vi "Extract Single Tone Information from Hann Spectrum.vi"(0 "complex spectrum in":cdb[](array[numeric]) format="%0.2f", 1 "time signal in":dbl[](array[numeric]) format="%0.2f", 5 "FFT size":i32, 7 "export mode":T2(ring), 9 "sampling frequency":dbl format="%0.2f", 11 "error in":errorcluster, 12 "advanced search":T3={"approx freq. (optional)"=-1.0, "search (+/- % of Fsampl.)"=5.0} {"search (+/- % of Fsampl.)" format="%0.2f"; "approx freq. (optional)" format="%0.2f"}) -> (3 "time signal out":dbl[](array[numeric]) format="%0.2p", 4 "complex spectrum out":cdb[](array[numeric]) format="%0.2f", 6 "detected frequency":dbl format="%0.3p", 8 "detected amplitude":dbl format="%0.3p", 10 "detected phase (deg)":dbl format="%0.3p", 14 "measurement info":T1 {"uncertainty" format="%0.2p"}, 15 "error out":errorcluster)   [LabVIEW 2020, in "NI_MAPro.lvlib"]
uses:
  NI_MAPro.lvlib
  NI_AALBase.lvlib
panel:
  # "Extract Single Tone Information\nfrom Hann weighted Spectrum"
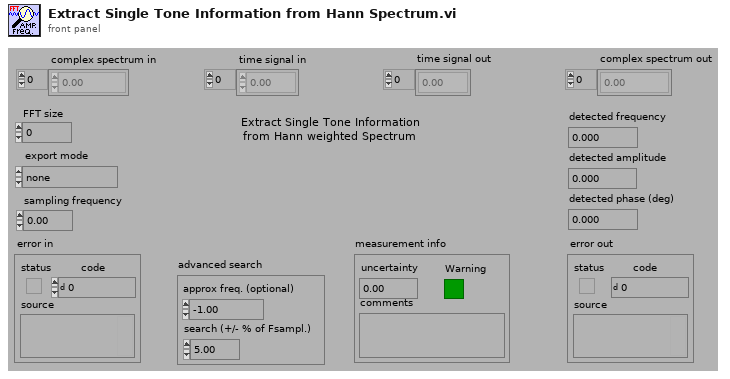
[diagram p1: front panel]
types:
  T1 = cluster{"uncertainty":dbl, "Warning":bool, "comments":string}
  T2 = enum32{"none", "input signal", "detected signal", "residual signal"}
  T3 = cluster{"approx freq. (optional)":dbl, "search (+/- % of Fsampl.)":dbl}
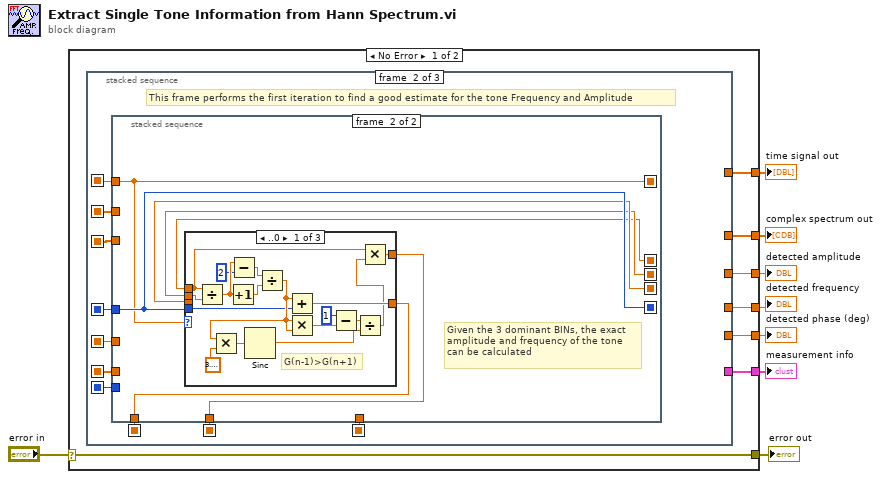
[diagram p0: block diagram]
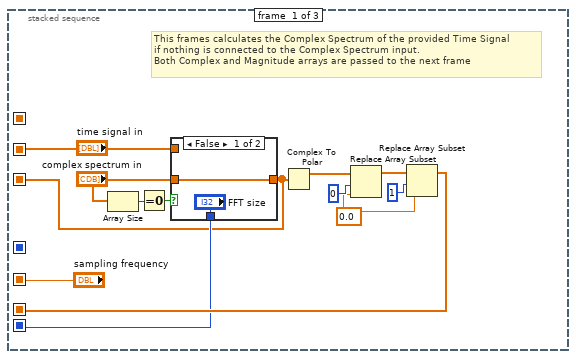
[diagram p2: hidden frame]
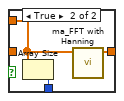
[diagram p3: hidden frame]
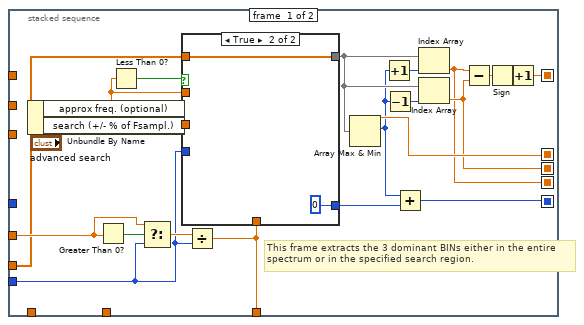
[diagram p4: hidden frame]
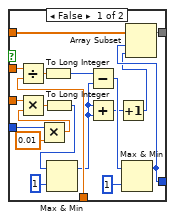
[diagram p5: hidden frame]
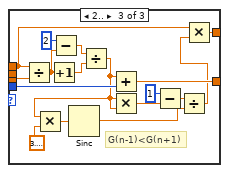
[diagram p7: hidden frame]
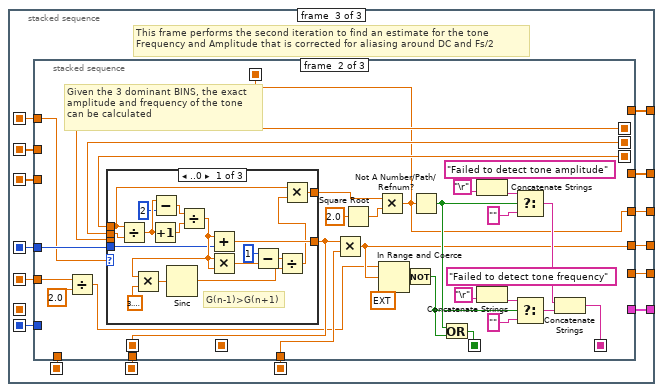
[diagram p8: hidden frame]
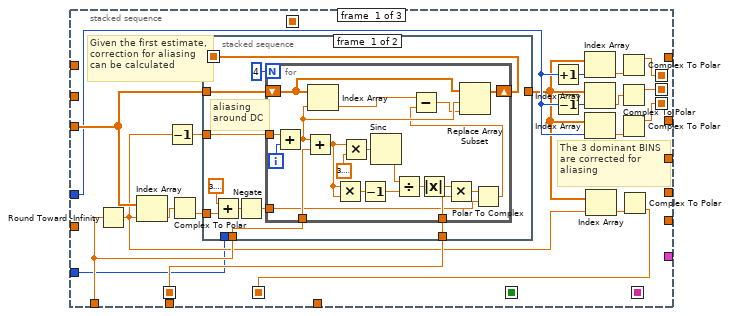
[diagram p9: hidden frame]
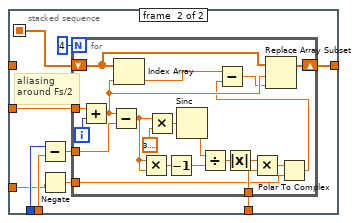
[diagram p10: hidden frame]
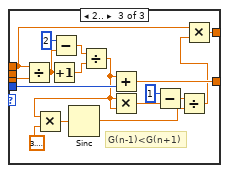
[diagram p12: hidden frame]
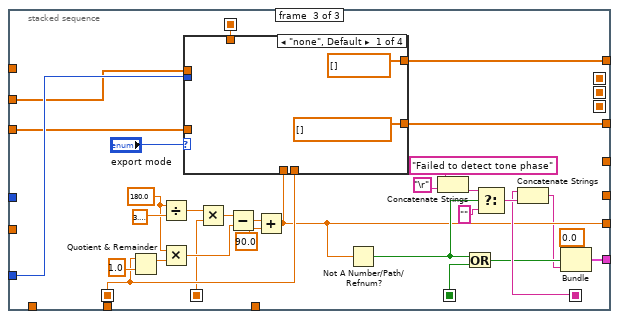
[diagram p13: hidden frame]
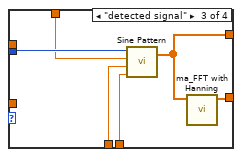
[diagram p15: hidden frame]
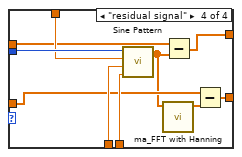
[diagram p16: hidden frame]
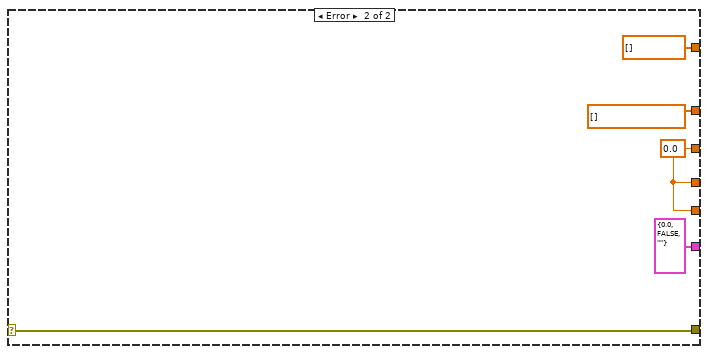
[diagram p17: hidden frame]
diagram:
  n1 = case shown="No Error" "error in" {
    selector: "error in" -> [w9 w343]
    tunnel: [w9 w343] -> w8
    tunnel: [w15 dbl[] [] ("Sinusoidal Pattern")] -> w7
    tunnel: [w14 cdb[] [] ("complex spectrum")] -> w6
    tunnel: [w13 w345] -> w5
    tunnel: [w12 w345] -> w4
    tunnel: [w11 w345] -> w3
    tunnel: [w10 cluster{dbl, bool, string} {0.0, FALSE, ""}] -> w2
    frame No Error {
      n2 = stacked-sequence {
        seq-local: ["time signal in" _ _] -> [_ w43 w140]
        seq-local: [w16 _ _] -> [_ w42 w139]
        seq-local: ["sampling frequency" _ _] -> [_ w41 w130]
        seq-local: [w25 _ _] -> [_ w40 _]
        seq-local: [w24 _ _] -> [_ w39 w141]
        seq-local: [_ w38 _] -> [_ _ w138]
        seq-local: [_ w37 _] -> [_ _ w143]
        seq-local: [_ w36 _] -> [_ _ w144]
        seq-local: [_ w35 _] -> [_ _ w137]
        seq-local: [_ w34 _] -> [_ _ w142]
        tunnel: [_ _ w136] -> w15
        tunnel: [_ _ w135] -> w14
        tunnel: [_ _ w134] -> w13
        tunnel: [_ _ w133] -> w12
        tunnel: [_ _ w132] -> w11
        tunnel: [_ _ w131] -> w10
        frame #0 {
          w20 = 0.0
          # "This frames calculates the Complex Spectrum of the provided Time Signal\nif nothing is connected to the Complex Spectrum input.\nBoth Complex and Magnitude arrays are passed to the next frame"
          n3 = Array Size(array="complex spectrum in") -> (size(s)=w18:i32)
          n4 = Equal To 0?(x=w18) -> (x = 0?=w17:bool)
          n5 = case shown="False" w17 {
            tunnel: [w30 w33] -> w16
            tunnel: "complex spectrum in" -> [w30 _]
            tunnel: "time signal in" -> [_ w32]
            tunnel: ["FFT size" w31] -> w24
            frame False {
            }
            frame True {
              n6 = Array Size(array=w32) -> (size(s)=w31:i32)
              n7 = call "ma_FFT with Hanning.vi"("time signal data"=w32) -> ("complex Hann spectrum"=w33:cdb[])  [unwired: 2 in, 8 out]
            }
          }
          n8 = Complex To Polar(r * e^(i*theta)=w16) -> (r=w23:dbl[])  [unwired: 1 out]
          n9 = Replace Array Subset(array=w23, new element=w20, index=0) -> (w22:dbl[])
          n10 = Replace Array Subset(array=w22, new element=w20, index=1) -> (w25:dbl[])
        }
        frame #1 {
          # "This frame performs the first iteration to find a good estimate for the tone Frequency and Amplitude"
          n11 = stacked-sequence {
            seq-local: [w58 _] -> [_ w90]
            seq-local: [w57 _] -> [_ w91]
            seq-local: [w56 _] -> [_ w92]
            seq-local: [w45 _] -> [_ w93]
            seq-local: [w55 _] -> [_ w87]
            tunnel: w43 -> [_ _]
            tunnel: w42 -> [_ _]
            tunnel: w41 -> [w50 _]
            tunnel: w40 -> [w49 _]
            tunnel: w39 -> [w48 _]
            tunnel: [_ w89] -> w38
            tunnel: [_ w93] -> w37
            tunnel: [w47 _] -> w36
            tunnel: [_ w88] -> w35
            tunnel: [_ w87] -> w34
            frame #0 {
              # "This frame extracts the 3 dominant BINs either in the entire\nspectrum or in the specified search region."
              n12 = Unbundle By Name("advanced search") -> ("approx freq. (optional)"=w52:dbl, "search (+/- % of Fsampl.)"=w65:dbl)
              n13 = Greater Than 0?(x=w50) -> (x > 0?=w53:bool)
              n14 = Less Than 0?(x=w52) -> (x < 0?=w63:bool)
              n15 = Select(t=w50, s=w53, f=w48) -> (s? t:f=w54:dbl)
              n16 = Divide(x=w54, y=w48) -> (x/y=w47:dbl)
              n17 = case shown="True" w63 {
                tunnel: [w74 w86] -> w64
                tunnel: w49 -> [w76 w86]
                tunnel: w48 -> [w84 _]
                tunnel: w65 -> [w82 _]
                tunnel: w47 -> [w79 _]
                tunnel: w52 -> [w80 _]
                tunnel: [w72 0] -> w44
                frame False {
                  n18 = Divide(x=w80, y=w79) -> (x/y=w78:dbl)
                  n19 = Multiply(x=w84, y=0.01) -> (x*y=w81:dbl)
                  n20 = Multiply(x=w82, y=w81) -> (x*y=w77:dbl)
                  n21 = To Long Integer(number=w78) -> (32bit integer=w75:i32)
                  n22 = To Long Integer(number=w77) -> (32bit integer=w67:i32)
                  n23 = Max & Min(x=w67, y=1 ("x")) -> (max(x,y)=w66:i32)  [unwired: 1 out]
                  n24 = Subtract(x=w75, y=w66) -> (x-y=w73:i32)
                  n25 = Add(x=w66, y=w66) -> (x+y=w70:i32)
                  n26 = Increment(x=w70) -> (x+1=w69:i32)
                  n27 = Max & Min(x=w73, y=1) -> (max(x,y)=w72:i32)  [unwired: 1 out]
                  n28 = Array Subset(array=w76, index=w72, length=w69) -> (w74:dbl[])
                }
                frame True {
                }
              }
              n29 = Array Max & Min(array=w64) -> (max value=w58:dbl, max index (indices)=w46:i32)  [unwired: 2 out]
              n30 = Increment(x=w46) -> (x+1=w59:i32)
              n31 = Decrement(x=w46) -> (x-1=w60:i32)
              n32 = Add(x=w46, y=w44) -> (x+y=w45:i32)
              n33 = Index Array(array=w64, index=w59) -> (element=w56:dbl)
              n34 = Index Array(array=w64, index=w60) -> (element=w57:dbl)
              n35 = Subtract(x=w56, y=w57) -> (x-y=w61:dbl)
              n36 = Sign(1:w61) -> (0:w62:dbl)
              n37 = Increment(x=w62) -> (x+1=w55:dbl)
            }
            frame #1 {
              # "Given the 3 dominant BINs, the exact\namplitude and frequency of the tone\ncan be calculated"
              n38 = case shown="..0" w87 {
                tunnel: w92 -> [_ _ w115]
                tunnel: w91 -> [w110 _ _]
                tunnel: w90 -> [w99 w111 w116]
                tunnel: [w107 w112 w125] -> w89
                tunnel: [w101 w111 w118] -> w88
                tunnel: w93 -> [w95 w112 w124]
                frame ..0 {
                  # "G(n-1)>G(n+1)"
                  n39 = Divide(x=w99, y=w110) -> (x/y=w97:dbl)
                  n40 = Increment(x=w97) -> (x+1=w108:dbl)
                  n41 = Subtract(x=w97, y=2) -> (x-y=w109:dbl)
                  n42 = Divide(x=w109, y=w108) -> (x/y=w104:dbl)
                  n43 = Multiply(x=w104, y=3.141592653589793) -> (x*y=w98:dbl)
                  n44 = Sinc(1:w98) -> (0:w94:dbl)
                  n45 = Add(x=w104, y=w95) -> (x+y=w107:dbl)
                  n46 = Multiply(x=w104, y=w104) -> (x*y=w103:dbl)
                  n47 = Subtract(x=1, y=w103) -> (x-y=w102:dbl)
                  n48 = Divide(x=w102, y=w94) -> (x/y=w100:dbl)
                  n49 = Multiply(x=w99, y=w100) -> (x*y=w101:dbl)
                }
                frame 1 {
                  # "G(n-1)=G(n+1)"
                }
                frame 2.. {
                  # "G(n-1)<G(n+1)"
                  n50 = Divide(x=w116, y=w115) -> (x/y=w128:dbl)
                  n51 = Increment(x=w128) -> (x+1=w126:dbl)
                  n52 = Subtract(x=2, y=w128) -> (x-y=w127:dbl)
                  n53 = Divide(x=w127, y=w126) -> (x/y=w121:dbl)
                  n54 = Multiply(x=w121, y=3.141592653589793) -> (x*y=w113:dbl)
                  n55 = Sinc(1:w113) -> (0:w114:dbl)
                  n56 = Add(x=w121, y=w124) -> (x+y=w125:dbl)
                  n57 = Multiply(x=w121, y=w121) -> (x*y=w120:dbl)
                  n58 = Subtract(x=1, y=w120) -> (x-y=w119:dbl)
                  n59 = Divide(x=w119, y=w114) -> (x/y=w117:dbl)
                  n60 = Multiply(x=w116, y=w117) -> (x*y=w118:dbl)
                }
              }
            }
          }
        }
        frame #2 {
          # "This frame performs the second iteration to find an estimate for the tone \nFrequency and Amplitude that is corrected for aliasing around DC and Fs/2"
          n61 = stacked-sequence {
            seq-local: [w155 _ _] -> [_ w252 _]
            seq-local: [w153 _ _] -> [_ w251 _]
            seq-local: [w151 _ _] -> [_ w250 _]
            seq-local: [_ w254 _] -> [_ _ w310]
            seq-local: [_ w227 _] -> [_ _ w316]
            seq-local: [w146 _ _] -> [_ _ w308]
            seq-local: [_ w237 _] -> [_ _ w300]
            seq-local: [_ w236 _] -> [_ _ w301]
            tunnel: w144 -> [_ w255 _]
            tunnel: w143 -> [w157 w253 _]
            tunnel: w142 -> [_ w249 _]
            tunnel: w141 -> [w145 _ w315]
            tunnel: w140 -> [_ _ w314]
            tunnel: w139 -> [w162 _ w313]
            tunnel: w138 -> [w160 _ _]
            tunnel: w137 -> [w150 _ _]
            tunnel: [_ _ w298] -> w136
            tunnel: [_ _ w297] -> w135
            tunnel: [_ _ w296] -> w134
            tunnel: [_ w235 _] -> w133
            tunnel: [_ w227 _] -> w132
            tunnel: [_ _ w292] -> w131
            tunnel: w130 -> [_ w231 _]
            frame #0 {
              # "The 3 dominant BINS\nare corrected for\naliasing"
              # "Given the first estimate,\ncorrection for aliasing\ncan be calculated"
              n62 = Round Toward -Infinity(1:w160) -> (0:w147:dbl)
              n63 = Index Array(array=w162, index=w147) -> (element=w163:cdb)
              n64 = Decrement(x=w147) -> (x-1=w164:dbl)
              n65 = Complex To Polar(r * e^(i*theta)=w163) -> (theta=w161:dbl)  [unwired: 1 out]
              n66 = stacked-sequence {
                seq-local: [w169 _] -> [_ w200]
                tunnel: w164 -> [w173 w203]
                tunnel: w162 -> [w172 _]
                tunnel: w161 -> [w168 w195]
                tunnel: w160 -> [w171 w198]
                tunnel: w150 -> [w170 w202]
                tunnel: [_ w201] -> w148
                tunnel: w145 -> [_ w197]
                frame #0 {
                  # "aliasing\naround DC"
                  n67 = Add(x=3.141592653589793, y=w168) -> (x+y=w166:dbl)
                  n68 = Negate(x=w166) -> (-x=w165:dbl)
                  n69 = for {
                    N: 4 -> [_]
                    tunnel: w173 -> [w194]
                    shift-right: [w179] -> w169
                    shift-left: w172 -> [w183]
                    tunnel: w171 -> [w192]
                    tunnel: w170 -> [w176]
                    tunnel: w165 -> [w175]
                    i -> [w193]
                    n70 = Add(x=w194, y=w193) -> (x+y=w184:dbl)
                    n71 = Add(x=w184, y=w192) -> (x+y=w185:dbl)
                    n72 = Index Array(array=w183, index=w184) -> (element=w181:cdb)
                    n73 = Multiply(x=w185, y=w185) -> (x*y=w189:dbl)
                    n74 = Multiply(x=w185, y=3.141592653589793) -> (x*y=w190:dbl)
                    n75 = Decrement(x=w189) -> (x-1=w187:dbl)
                    n76 = Sinc(1:w190) -> (0:w188:dbl)
                    n77 = Divide(x=w188, y=w187) -> (x/y=w186:dbl)
                    n78 = Absolute Value(x=w186) -> (abs(x)=w178:dbl)
                    n79 = Multiply(x=w178, y=w176) -> (x*y=w177:dbl)
                    n80 = Polar To Complex(1:w175, 2:w177) -> (0:w180:cdb)
                    n81 = Subtract(x=w181, y=w180) -> (x-y=w182:cdb)
                    n82 = Replace Array Subset(array=w183, new element=w182, index=w184) -> (w179:cdb[])
                  }
                }
                frame #1 {
                  # "aliasing\naround Fs/2"
                  n83 = Subtract(x=w197, y=w198) -> (x-y=w199:dbl)
                  n84 = Negate(x=w195) -> (-x=w196:dbl)
                  n85 = for {
                    N: 4 -> [_]
                    tunnel: w203 -> [w224]
                    shift-right: [w211] -> w201
                    shift-left: w200 -> [w215]
                    tunnel: w202 -> [w208]
                    tunnel: w199 -> [w206]
                    tunnel: w196 -> [w205]
                    i -> [w223]
                    n86 = Add(x=w224, y=w223) -> (x+y=w216:dbl)
                    n87 = Subtract(x=w216, y=w206) -> (x-y=w207:dbl)
                    n88 = Index Array(array=w215, index=w216) -> (element=w213:cdb)
                    n89 = Multiply(x=w207, y=w207) -> (x*y=w220:dbl)
                    n90 = Multiply(x=w207, y=3.141592653589793) -> (x*y=w221:dbl)
                    n91 = Decrement(x=w220) -> (x-1=w218:dbl)
                    n92 = Sinc(1:w221) -> (0:w219:dbl)
                    n93 = Divide(x=w219, y=w218) -> (x/y=w217:dbl)
                    n94 = Absolute Value(x=w217) -> (abs(x)=w210:dbl)
                    n95 = Multiply(x=w210, y=w208) -> (x*y=w209:dbl)
                    n96 = Polar To Complex(1:w205, 2:w209) -> (0:w212:cdb)
                    n97 = Subtract(x=w213, y=w212) -> (x-y=w214:cdb)
                    n98 = Replace Array Subset(array=w215, new element=w214, index=w216) -> (w211:cdb[])
                  }
                }
              }
              n99 = Increment(x=w157) -> (x+1=w158:i32)
              n100 = Decrement(x=w157) -> (x-1=w159:i32)
              n101 = Index Array(array=w148, index=w158) -> (element=w152:cdb)
              n102 = Index Array(array=w148, index=w159) -> (element=w154:cdb)
              n103 = Index Array(array=w148, index=w157) -> (element=w156:cdb)
              n104 = Index Array(array=w148, index=w147) -> (element=w149:cdb)
              n105 = Complex To Polar(r * e^(i*theta)=w152) -> (r=w151:dbl)  [unwired: 1 out]
              n106 = Complex To Polar(r * e^(i*theta)=w154) -> (r=w153:dbl)  [unwired: 1 out]
              n107 = Complex To Polar(r * e^(i*theta)=w156) -> (r=w155:dbl)  [unwired: 1 out]
              n108 = Complex To Polar(r * e^(i*theta)=w149) -> (theta=w146:dbl)  [unwired: 1 out]
            }
            frame #1 {
              # "Given the 3 dominant BINS, the exact\namplitude and frequency of the tone\ncan be calculated"
              n109 = Divide(x=w231, y=2.0) -> (x/y=w229:dbl)
              n110 = case shown="..0" w249 {
                tunnel: w250 -> [_ _ w277]
                tunnel: w251 -> [w272 _ _]
                tunnel: w252 -> [w261 w273 w278]
                tunnel: [w269 w274 w287] -> w254
                tunnel: [w263 w273 w280] -> w226
                tunnel: w253 -> [w257 w274 w286]
                frame ..0 {
                  # "G(n-1)>G(n+1)"
                  n111 = Divide(x=w261, y=w272) -> (x/y=w259:dbl)
                  n112 = Increment(x=w259) -> (x+1=w270:dbl)
                  n113 = Subtract(x=w259, y=2) -> (x-y=w271:dbl)
                  n114 = Divide(x=w271, y=w270) -> (x/y=w266:dbl)
                  n115 = Multiply(x=w266, y=3.141592653589793) -> (x*y=w260:dbl)
                  n116 = Sinc(1:w260) -> (0:w256:dbl)
                  n117 = Add(x=w266, y=w257) -> (x+y=w269:dbl)
                  n118 = Multiply(x=w266, y=w266) -> (x*y=w265:dbl)
                  n119 = Subtract(x=1, y=w265) -> (x-y=w264:dbl)
                  n120 = Divide(x=w264, y=w256) -> (x/y=w262:dbl)
                  n121 = Multiply(x=w261, y=w262) -> (x*y=w263:dbl)
                }
                frame 1 {
                  # "G(n-1)=G(n+1)"
                }
                frame 2.. {
                  # "G(n-1)<G(n+1)"
                  n122 = Divide(x=w278, y=w277) -> (x/y=w290:dbl)
                  n123 = Increment(x=w290) -> (x+1=w288:dbl)
                  n124 = Subtract(x=2, y=w290) -> (x-y=w289:dbl)
                  n125 = Divide(x=w289, y=w288) -> (x/y=w283:dbl)
                  n126 = Multiply(x=w283, y=3.141592653589793) -> (x*y=w275:dbl)
                  n127 = Sinc(1:w275) -> (0:w276:dbl)
                  n128 = Add(x=w283, y=w286) -> (x+y=w287:dbl)
                  n129 = Multiply(x=w283, y=w283) -> (x*y=w282:dbl)
                  n130 = Subtract(x=1, y=w282) -> (x-y=w281:dbl)
                  n131 = Divide(x=w281, y=w276) -> (x/y=w279:dbl)
                  n132 = Multiply(x=w278, y=w279) -> (x*y=w280:dbl)
                }
              }
              n133 = Multiply(x=w254, y=w255) -> (x*y=w235:dbl)
              n134 = Square Root(x=2.0) -> (sqrt(x)=w225:dbl)
              n135 = Multiply(x=w226, y=w225) -> (x*y=w227:dbl)
              n136 = In Range and Coerce(upper limit=w229, x=w235, lower limit=ext 0.0 ("lo")) -> (In Range?=w233:bool)  [unwired: 1 out]
              n137 = Not(x=w233) -> (.not. x?=w232:bool)
              n138 = Not A Number/Path/Refnum?(number/path/refnum=w227) -> (NaN/Path/Refnum?=w238:bool)
              n139 = Or(x=w238, y=w232) -> (x .or. y?=w237:bool)
              n140 = Concatenate Strings("Failed to detect tone amplitude", "\r") -> (w246:string)
              n141 = Concatenate Strings("Failed to detect tone frequency", "\r") -> (w243:string)
              n142 = Select(t=w246, s=w238, f="") -> (s? t:f=w239:string)
              n143 = Select(t=w243, s=w232, f="") -> (s? t:f=w240:string)
              n144 = Concatenate Strings(w239, w240) -> (w236:string)
            }
            frame #2 {
              w307 = 180.0 ("x")
              n145 = Quotient & Remainder(x=w310, y=1.0) -> (x-y*floor(x/y)=w309:dbl)  [unwired: 1 out]
              n146 = Divide(x=w307, y=3.141592653589793) -> (x/y=w317:dbl)
              n147 = Multiply(x=w307, y=w309) -> (x*y=w321:dbl)
              n148 = Multiply(x=w317, y=w308) -> (x*y=w319:dbl)
              n149 = Subtract(x=w319, y=w321) -> (x-y=w320:dbl)
              n150 = Add(x=w320, y=90.0) -> (x+y=w296:dbl)
              n151 = case shown="\"none\", Default" "export mode" {
                tunnel: w296 -> [_ _ w332 w342]
                tunnel: w315 -> [_ _ w331 w341]
                tunnel: [dbl[] [] ("Sinusoidal Pattern") w326 w328 w337] -> w298
                tunnel: w310 -> [_ _ w330 w340]
                tunnel: w316 -> [_ _ w329 w339]
                tunnel: w314 -> [_ w326 _ w338]
                tunnel: [cdb[] [] ("complex spectrum out") w325 w327 w336] -> w297
                tunnel: w313 -> [_ w325 _ w335]
                frame "none", Default {
                }
                frame "input signal" {
                }
                frame "detected signal" {
                  n152 = call "Sine Pattern.vi"("cycles"=w330, "phase(degrees)"=w332, "amplitude"=w329, "samples"=w331) -> ("Sinusoidal Pattern"=w328:dbl[])  [unwired: 1 out]
                  n153 = call "ma_FFT with Hanning.vi"("time signal data"=w328) -> ("complex Hann spectrum"=w327:cdb[])  [unwired: 2 in, 8 out]
                }
                frame "residual signal" {
                  n154 = call "Sine Pattern.vi"("cycles"=w340, "phase(degrees)"=w342, "amplitude"=w339, "samples"=w341) -> ("Sinusoidal Pattern"=w333:dbl[])  [unwired: 1 out]
                  n155 = call "ma_FFT with Hanning.vi"("time signal data"=w333) -> ("complex Hann spectrum"=w334:cdb[])  [unwired: 2 in, 8 out]
                  n156 = Subtract(x=w338, y=w333) -> (x-y=w337:dbl[])
                  n157 = Subtract(x=w335, y=w334) -> (x-y=w336:cdb[])
                }
              }
              n158 = Not A Number/Path/Refnum?(number/path/refnum=w296) -> (NaN/Path/Refnum?=w299:bool)
              n159 = Concatenate Strings("Failed to detect tone phase", "\r") -> (w303:string)
              n160 = Or(x=w299, y=w300) -> (x .or. y?=w295:bool)
              n161 = Select(t=w303, s=w299, f="") -> (s? t:f=w306:string)
              n162 = Concatenate Strings(w301, w306) -> (w294:string)
              n163 = Bundle(0.0, w295, w294) -> (w292:cluster{dbl, bool, string})  [unwired: 1 out]
            }
          }
        }
      }
    }
    frame Error {
      w345 = 0.0
    }
  }
  "error out" <- w8
  "measurement info" <- w2
  "complex spectrum out" <- w6
  "time signal out" <- w7
  "detected phase (deg)" <- w5
  "detected frequency" <- w4
  "detected amplitude" <- w3
